vi "TDMSFileViewerLocalizedText.vi"() -> ()   [LabVIEW 2009]
panel:
  in  "False":string="false"
  in  "True":string="true"
  in  "pattern label tdm":string="National Instruments TDM"
  in  "prompt tdm":string="Open TDM File"
  in  "Loaded values %d ... %d":string="Loaded values %d ... %d"
  in  "pattern label tdms":string="National Instruments TDM Streaming"
  in  "prompt tdms":string="Open TDMS File"
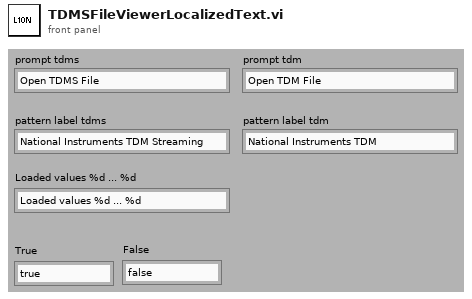
[diagram p1: front panel]
diagram:
